vi "Set Hardware Manager.vi"(8 "error in (no error)":errorcluster, 10 "HardwareManager":refnum<class "HardwareManager.lvclass">=refnum, 11 "Base Step in":refnum<class "Base Step.lvclass">) -> (0 "error out":errorcluster, 3 "Base Step out":refnum<class "Base Step.lvclass">)   [LabVIEW 2020]
uses:
  Base Step.lvclass
  HardwareManager/HardwareManager.lvclass
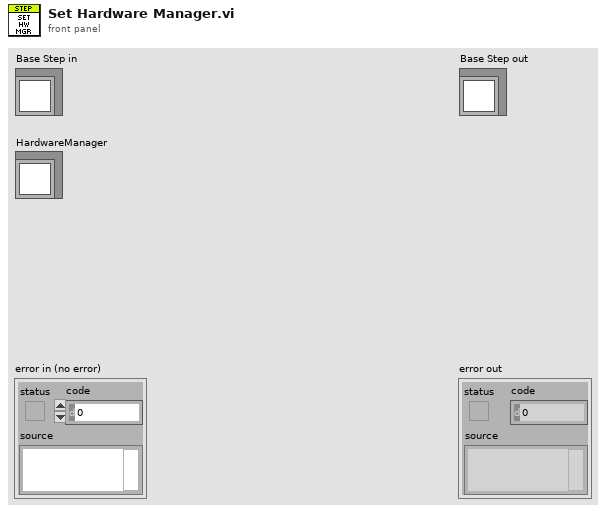
[diagram p1: front panel]
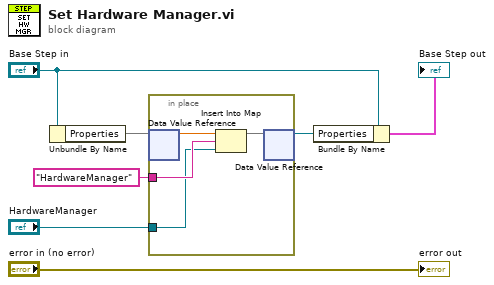
[diagram p0: block diagram]
diagram:
  n1 = Unbundle By Name("Base Step in") -> ("Properties"=w4)
  n2 = in-place {
    in-place-border: "HardwareManager" ("Key") -> [w11]
    in-place-border: "HardwareManager" -> [w10]
    n3 = in-place-dvr #1(w4) -> (w9:dbl)  [unwired: 1 out]
    n4 = Insert Into Map(map in=w9, key=w11, value=w10) -> (map out=w8:map{string, i32})  [unwired: 2 out]
    n5 = in-place-dvr #1(w8) -> (w3:refnum<data-value>)  [unwired: 1 out]
  }
  n6 = Bundle By Name(cluster="Base Step in", "Properties"=w3) -> (→"Base Step out":cluster{})
  "error out" <- "error in (no error)"
